vi "Clear HW Torque Trim Sensors 4 and 5.vi"(6 "error in":errorcluster, 8 "MaxRead":i32, 9 "Channel in":u16) -> (0 "error out":errorcluster, 1 "Messages":T1(array[cluster]) {"DATA[1]" format="%.0x"; "DATA[3]" format="%.0x"; "DATA[4]" format="%.0x"}, 2 "Pass":bool, 3 "Channel out":u16)   [LabVIEW 2023]
uses:
  4f930f32-d09a-43ef-bca1-8b214b378bd5.vi
  ca49bb01-4f9d-4fc6-af7c-560520f89dfa.vi
  e8470de1-fa2d-4ee3-b50e-96bd89dc731f.vi
  d0f02419-cfb7-4a5e-bc3c-f035efdb0e96.vi
  Communication/PCAN2023/PCAN API.lvlib
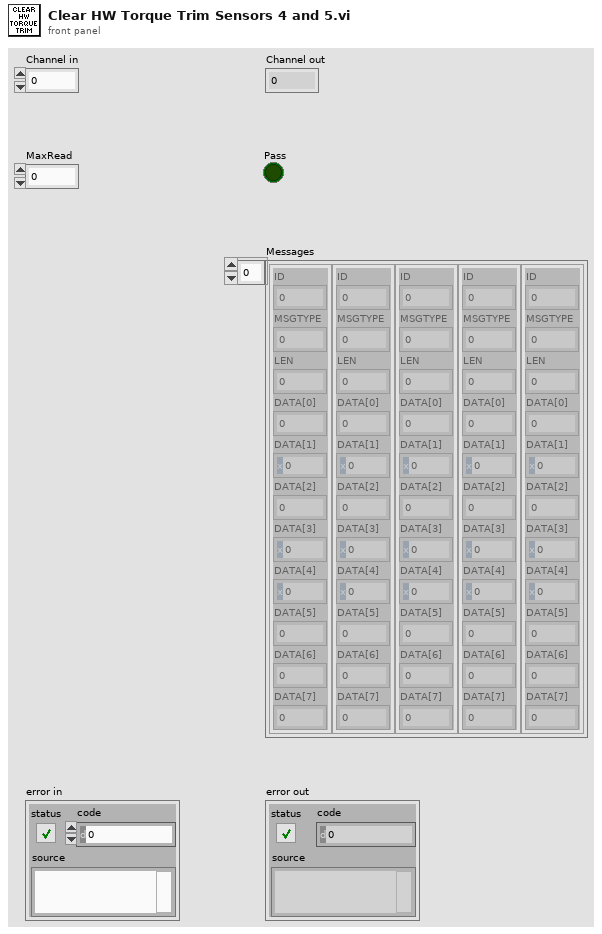
[diagram p1: front panel]
types:
  T1 = cluster{"ID":u32, "MSGTYPE":u8, "LEN":u8, "DATA[0]":u8, "DATA[1]":u8, "DATA[2]":u8, "DATA[3]":u8, "DATA[4]":u8, "DATA[5]":u8, "DATA[6]":u8, "DATA[7]":u8}[]
  T2 = cluster{"ID":u32, "MSGTYPE":u8, "LEN":u8, "DATA[0]":u8, "DATA[1]":u8, "DATA[2]":u8, "DATA[3]":u8, "DATA[4]":u8, "DATA[5]":u8, "DATA[6]":u8, "DATA[7]":u8}
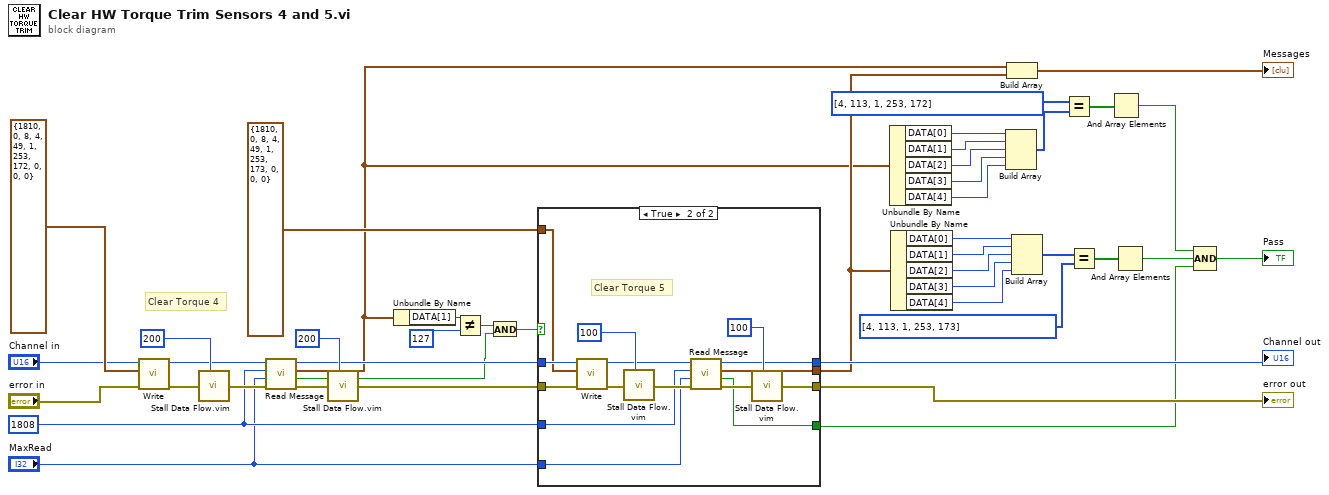
[diagram p0: block diagram]
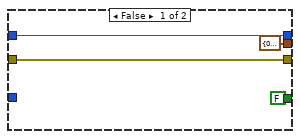
[diagram p2: hidden frame]
diagram:
  w4 = u32 1808 ("ID")
  # "Clear Torque 4"
  n1 = call "Write.vi"("error in"="error in", "MessageBuffer"=T2 {"ID"=1810, "MSGTYPE"=0, "LEN"=8, "DATA[0]"=4, "DATA[1]"=49, "DATA[2]"=1, "DATA[3]"=253, "DATA[4]"=172, "DATA[5]"=0, "DATA[6]"=0, "DATA[7]"=0}, "Channel"="Channel in") -> ("error out"=w40:errorcluster, "Channel out"=w12:u16)  [unwired: 5 in, 2 out]
  n2 = call "Stall Data Flow.vim"("value in"=w40, "milliseconds to wait"=u32 200) -> ("value out"=w10:errorcluster)  [unwired: 1 out]
  n3 = call "Read Message.vi"("error in"=w10, "MaxRead"="MaxRead", "ID"=w4, "Channel in"=w12) -> ("error out"=w9:errorcluster, "Passed"=w6:bool, "Last Message"=w8:T2, "Channel out"=w11:u16)  [unwired: 3 in, 1 out]
  n4 = call "Stall Data Flow.vim"("value in"=w9, "milliseconds to wait"=u32 200) -> ("value out"=w21:errorcluster)  [unwired: 1 out]
  n5 = Unbundle By Name(w8) -> ("DATA[1]"=w36:u8)
  n6 = Not Equal?(x=w36, y=u8 127) -> (x != y?=w7:bool)
  n7 = And(x=w7, y=w6) -> (x .and. y?=w5:bool)
  n8 = case shown="True" w5 {
    tunnel: w11 -> [w47 w63]
    tunnel: w21 -> [w45 w62]
    tunnel: [w45 w61] -> w39
    tunnel: [FALSE w51] -> w1
    tunnel: [w47 w55] -> w38
    tunnel: T2 {"ID"=1810, "MSGTYPE"=0, "LEN"=8, "DATA[0]"=4, "DATA[1]"=49, "DATA[2]"=1, "DATA[3]"=253, "DATA[4]"=173, "DATA[5]"=0, "DATA[6]"=0, "DATA[7]"=0} ("MessageBuffer") -> [_ w60]
    tunnel: [T2 {"ID"=0, "MSGTYPE"=0, "LEN"=0, "DATA[0]"=0, "DATA[1]"=0, "DATA[2]"=0, "DATA[3]"=0, "DATA[4]"=0, "DATA[5]"=0, "DATA[6]"=0, "DATA[7]"=0} w52] -> w19
    tunnel: w4 -> [_ w50]
    tunnel: "MaxRead" -> [_ w49]
    frame False {
    }
    frame True {
      # "Clear Torque 5"
      n9 = call "Write.vi"("error in"=w62, "MessageBuffer"=w60, "Channel"=w63) -> ("error out"=w58:errorcluster, "Channel out"=w56:u16)  [unwired: 5 in, 2 out]
      n10 = call "Stall Data Flow.vim"("value in"=w58, "milliseconds to wait"=u32 100) -> ("value out"=w54:errorcluster)  [unwired: 1 out]
      n11 = call "Read Message.vi"("error in"=w54, "MaxRead"=w49, "ID"=w50, "Channel in"=w56) -> ("error out"=w53:errorcluster, "Passed"=w51:bool, "Last Message"=w52:T2, "Channel out"=w55:u16)  [unwired: 3 in, 1 out]
      n12 = call "Stall Data Flow.vim"("value in"=w53, "milliseconds to wait"=u32 100) -> ("value out"=w61:errorcluster)  [unwired: 1 out]
    }
  }
  "error out" <- w39
  "Channel out" <- w38
  n13 = Unbundle By Name(w8) -> ("DATA[0]"=w25:u8, "DATA[1]"=w24:u8, "DATA[2]"=w23:u8, "DATA[3]"=w17:u8, "DATA[4]"=w16:u8)
  n14 = Unbundle By Name(w19) -> ("DATA[0]"=w33:u8, "DATA[1]"=w32:u8, "DATA[2]"=w31:u8, "DATA[3]"=w30:u8, "DATA[4]"=w29:u8)
  n15 = Build Array(w25, w24, w23, w17, w16) -> (w14:u8[])
  n16 = Build Array(w8, w19) -> (→"Messages":T1)
  n17 = Build Array(w33, w32, w31, w30, w29) -> (w28:u8[])
  n18 = Equal?(x=u8[] [4, 113, 1, 253, 172] ("y"), y=w14) -> (x = y?=w13:bool[])
  n19 = Equal?(x=w28, y=u8[] [4, 113, 1, 253, 173]) -> (x = y?=w26:bool[])
  n20 = And Array Elements(Boolean array=w13) -> (logical AND=w2:bool)
  n21 = And Array Elements(Boolean array=w26) -> (logical AND=w18:bool)
  n22 = Compound Arithmetic op=AND(w2, w18, w1) -> (→"Pass":bool)
